vi "总氮流程质控自动启动.vi"(10 "总氮量程切换":enum32{"H", "L", "AUTO"}(ring)=enum."AUTO", 11 "参数":T1={"是否启用仪器"=FALSE, "CODMn"={"启动测量模式"={"测量模式"=enum."水样测量"}, "确定按钮"=TRUE}, "启动模块"={"氨氮"=FALSE, "总磷"=FALSE, "总氮"=FALSE, "COD"=FALSE}, "常规启动"=FALSE, "直接启动"=FALSE}) -> ()   [LabVIEW 2016, in "质控单元.lvlib"]
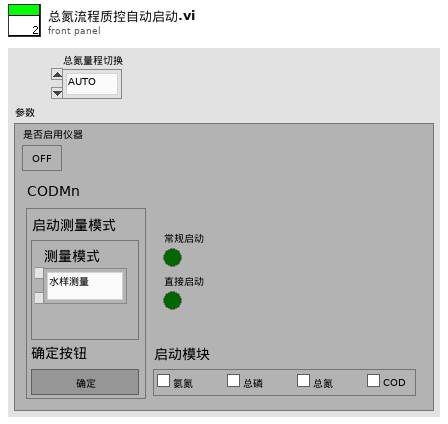
[diagram p1: front panel]
types:
  T1 = cluster{"是否启用仪器":bool, "CODMn":cluster{"启动测量模式":cluster{"测量模式":enum16{"水样测量", "标样核查", "加标回收", "平行样", "校零", "校标"}}, "确定按钮":bool}, "启动模块":cluster{"氨氮":bool, "总磷":bool, "总氮":bool, "COD":bool}, "常规启动":bool, "直接启动":bool}
  T2 = cluster{"R0":i16, "R1":i16, "R2":i16, "R3":i16, "R4":i16, "R5":i16, "R6":i16, "R7":i16, "R8":i16, "R9":i16, "R10":i16, "R11":i16, "R12":i16, "R13":i16, "R14":i16, "R15":i16, "R16":i16, "R17":i16, "R18":i16, "R19":i16, "R20":i16, "R21":i16, "R22":i16, "R23":i16, "R24":i16, "R25":i16, "R26":i16, "R27":i16, "R28":i16, "R29":i16, "R30":i16, "R31":i16, "R32":i16, "R33":i16, "R34":i16, "R35":i16, "R36":i16, "R37":i16, "R38":i16, "R39":i16, "R40":i16, "R41":i16, "R42":i16, "R43":i16, "R44":i16, "R45":i16, "R46":i16, "R47":i16, "R48":i16, "R49":i16, "R50":i16, "R51":i16, "R52":i16, "R53":i16, "R54":i16, "R55":i16, "R56":i16}
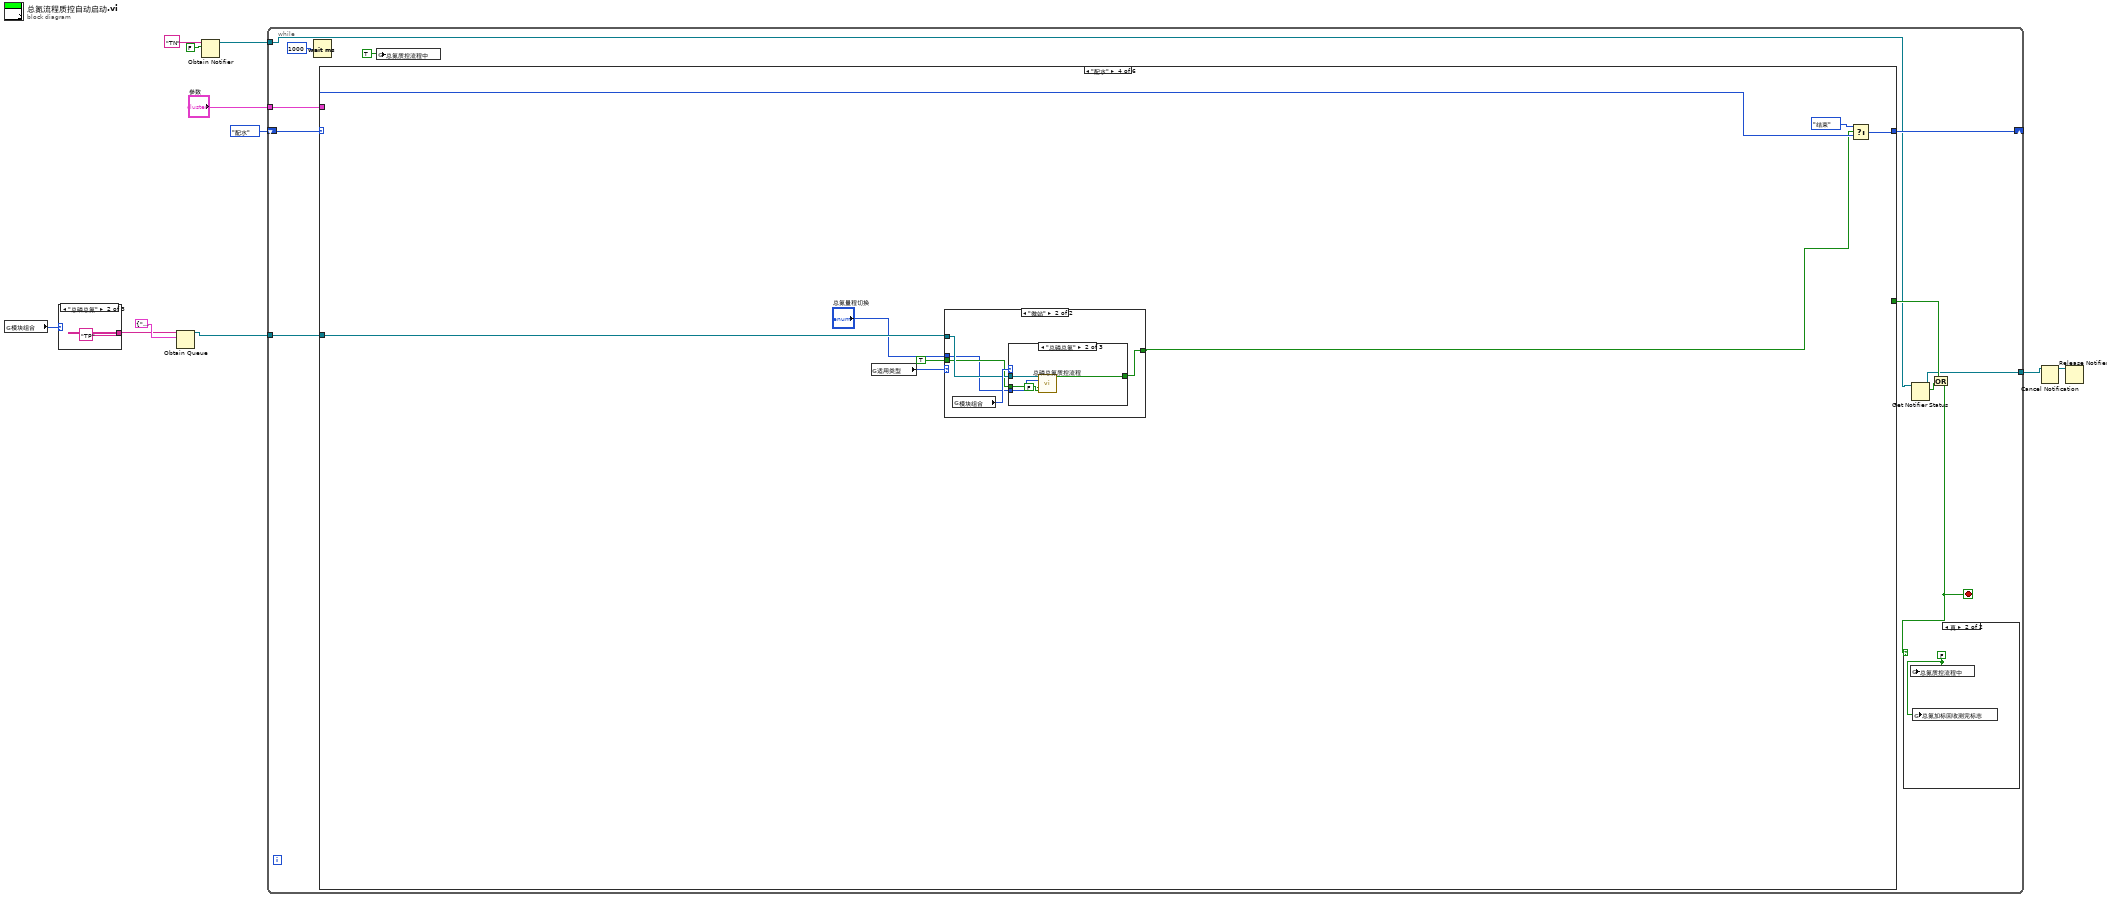
[diagram p0: block diagram]
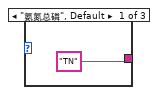
[diagram p2: hidden frame]
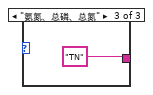
[diagram p3: hidden frame]
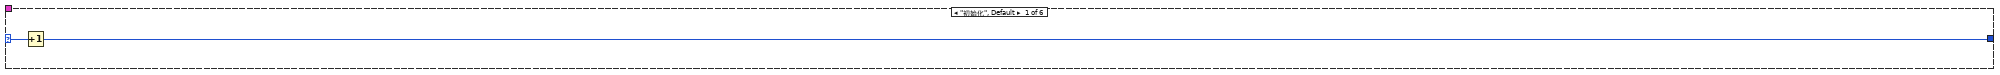
[diagram p5: hidden frame]
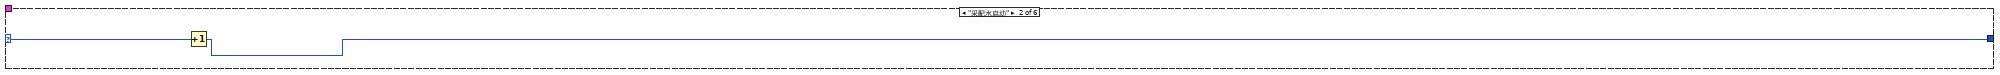
[diagram p6: hidden frame]
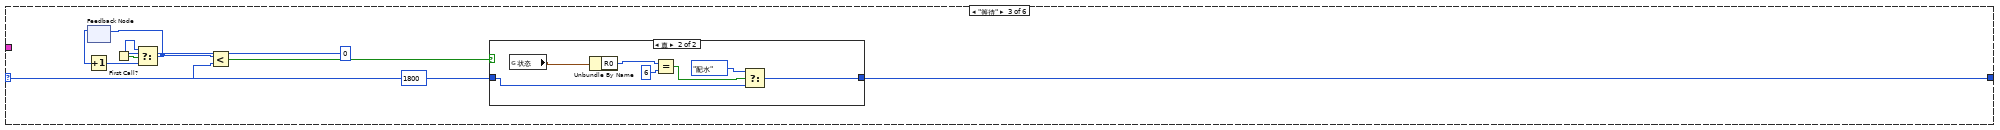
[diagram p7: hidden frame]
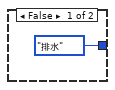
[diagram p8: hidden frame]
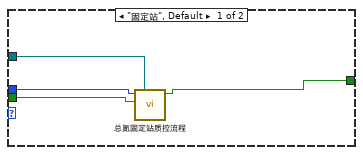
[diagram p9: hidden frame]
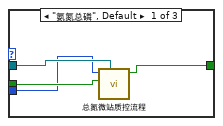
[diagram p10: hidden frame]
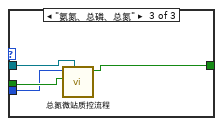
[diagram p11: hidden frame]
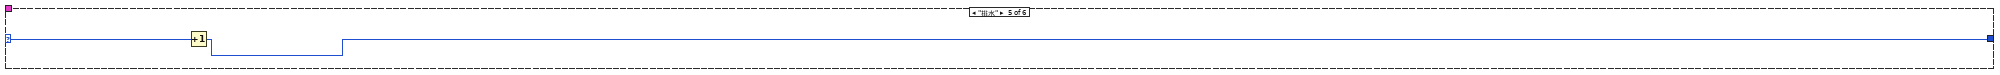
[diagram p12: hidden frame]
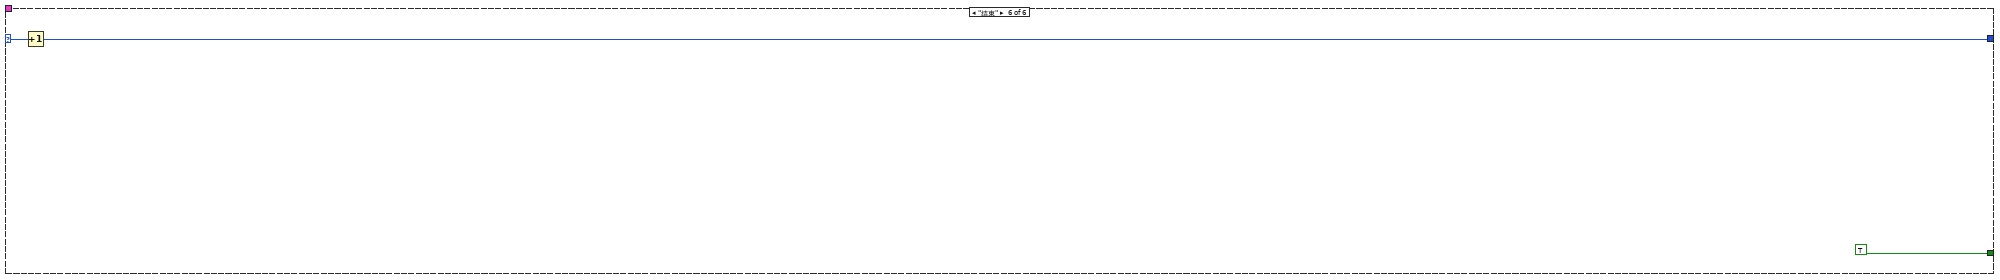
[diagram p13: hidden frame]
diagram:
  n1 = global read "断电保存全局.vi" "模块组合"() -> (w2:enum16{"氨氮总磷", "总磷总氮", "氨氮、总磷、总氮"})
  n2 = case shown="\"总磷总氮\"" w2 {
    tunnel: ["TN" ("名称（未命名）") "TP" ("名称（未命名）") "TN" ("名称（未命名）")] -> w1
    frame "氨氮总磷", Default {
    }
    frame "总磷总氮" {
    }
    frame "氨氮、总磷、总氮" {
    }
  }
  n3 = Obtain Queue(name (unnamed)=w1, element data type=cluster{"命令":string, "data":variant} {"命令"="", "data"=variant}) -> (queue out=w3:refnum<queue>)  [unwired: 3 in, 2 out]
  n4 = Obtain Notifier(name (unnamed)="TN" ("名称（未命名）"), notification data type=FALSE) -> (notifier out=w7:refnum<notifier>)  [unwired: 2 in, 2 out]
  n5 = while {
    shift-right: [w24] -> _
    shift-left: enum16{"初始化", "采配水启动", "等待", "配水", "排水", "结束"}."配水" ("枚举") -> [w25]
    tunnel: "参数" -> [w22]
    tunnel: w3 -> [w21]
    tunnel: w7 -> [w19]
    tunnel: [w17] -> w5
    stop <- w15 stop-if-true
    n6 = Wait (ms)(milliseconds to wait=u32 1000 ("等待时间（毫秒）")) -> ()  [unwired: 1 out]
    n7 = case shown="\"配水\"" w25 {
      selector: w25 -> [w28 w30 w37 w54 w79 w82]
      tunnel: [w27 w29 w36 w53 w78 w81] -> w24
      tunnel: [_ _ _ _ _ TRUE] -> w20
      tunnel: w22 -> [_ _ _ _ _ _]
      tunnel: w21 -> [_ _ _ w50 _ _]
      frame "初始化", Default {
        n8 = Increment(x=w28) -> (x+1=w27:enum16{"初始化", "采配水启动", "等待", "配水", "排水", "结束"})
      }
      frame "采配水启动" {
        n9 = Increment(x=w30) -> (x+1=w29:enum16{"初始化", "采配水启动", "等待", "配水", "排水", "结束"})
      }
      frame "等待" {
        n10 = feedback #1() -> (w33:i32)  [unwired: 1 in]
        n11 = Increment(x=w33) -> (x+1=w32:i32)
        n12 = First Call?() -> (First Call?: T/F=w34:bool)
        n13 = Select(t=0, s=w34, f=w32) -> (s? t:f=w31:i32)
        n14 = feedback-in #1(w31) -> ()
        n15 = Less?(x=w31, y=1800) -> (x < y?=w38:bool)
        n16 = case shown="真" w38 {
          tunnel: w37 -> [_ w43]
          tunnel: [enum16{"初始化", "采配水启动", "等待", "配水", "排水", "结束"}."排水" ("枚举") w42] -> w36
          frame False {
          }
          frame True {
            n17 = global read "与采配水交互全局.vi" "状态"() -> (w41:T2)
            n18 = Unbundle By Name(w41) -> ("R0"=w47:i16)
            n19 = Equal?(x=w47, y=i16 6) -> (x = y?=w45:bool)
            n20 = Select(t=enum16{"初始化", "采配水启动", "等待", "配水", "排水", "结束"}."配水" ("枚举"), s=w45, f=w43) -> (s? t:f=w42:enum16{"初始化", "采配水启动", "等待", "配水", "排水", "结束"})
          }
        }
      }
      frame "配水" {
        n21 = global read "断电保存全局.vi" "适用类型"() -> (w51:enum16{"固定站", "微站"})
        n22 = case shown="\"微站\"" w51 {
          tunnel: w50 -> [w59 w63]
          tunnel: "总氮量程切换" -> [w58 w61]
          tunnel: TRUE ("氨氮") -> [w57 w62]
          tunnel: [w56 w60] -> w49
          frame "固定站", Default {
            n23 = call "总氮固定站质控流程.vi"("队列输入TN"=w59, "总氮"=w57, "总氮量程切换"=w58) -> ("布尔"=w56:bool)  [unwired: 7 in]
          }
          frame "微站" {
            n24 = global read "断电保存全局.vi" "模块组合"() -> (w64:enum16{"氨氮总磷", "总磷总氮", "氨氮、总磷、总氮"})
            n25 = case shown="\"总磷总氮\"" w64 {
              tunnel: w63 -> [w68 w73 w77]
              tunnel: w62 -> [w67 w71 w76]
              tunnel: w61 -> [w66 w70 w75]
              tunnel: [w65 w72 w74] -> w60
              frame "氨氮总磷", Default {
                n26 = call "总氮微站质控流程.vi"("队列输入TN"=w68, "总氮"=w67, "总氮量程切换"=w66) -> ("布尔"=w65:bool)  [unwired: 7 in]
              }
              frame "总磷总氮" {
                n27 = call "总磷总氮质控流程.vi"("队列输入TP"=w73, "总氮量程切换"=w70, "总磷"=FALSE, "总氮"=w71) -> ("布尔"=w72:bool)  [unwired: 9 in, 2 out]
              }
              frame "氨氮、总磷、总氮" {
                n28 = call "总氮微站质控流程.vi"("队列输入TN"=w77, "总氮"=w76, "总氮量程切换"=w75) -> ("布尔"=w74:bool)  [unwired: 7 in]
              }
            }
          }
        }
        n29 = Select(t=enum16{"初始化", "采配水启动", "等待", "配水", "排水", "结束"}."结束" ("枚举"), s=w49, f=w54) -> (s? t:f=w53:enum16{"初始化", "采配水启动", "等待", "配水", "排水", "结束"})
      }
      frame "排水" {
        n30 = Increment(x=w79) -> (x+1=w78:enum16{"初始化", "采配水启动", "等待", "配水", "排水", "结束"})
      }
      frame "结束" {
        n31 = Increment(x=w82) -> (x+1=w81:enum16{"初始化", "采配水启动", "等待", "配水", "排水", "结束"})
      }
    }
    n32 = global write "质控测完标志全局 1.vi" "总氮质控流程中"(TRUE ("氨氮质控流程中")) -> ()
    n33 = Get Notifier Status(notifier=w19) -> (notifier out=w17:refnum<notifier>, current notification=w18:bool)  [unwired: 1 in, 3 out]
    n34 = Or(x=w20, y=w18) -> (x .or. y?=w15:bool)
    n35 = case shown="真" w15 {
      frame False {
      }
      frame True {
        w26 = FALSE ("氨氮质控流程中")
        n36 = global write "质控测完标志全局 1.vi" "总氮质控流程中"(w26) -> ()
        n37 = global write "质控测完标志全局 1.vi" "总氮加标回收测完标志"(w26) -> ()
      }
    }
  }
  n38 = Cancel Notification(0:w5) -> (8:w6:refnum<notifier>)  [unwired: 1 in, 2 out]
  n39 = Release Notifier(notifier=w6) -> ()  [unwired: 2 in, 3 out]
